vi "setTensao.vi"(6 "delay(ms)":dbl, 7 "Ponto atual":i32, 8 "T.M":dbl caption="Tensão máxima", 9 "P.D.J":dbl, 10 "T.J":dbl caption="Tensão\ndo joelho", 11 "P.A.J":dbl) -> (3 "output voltage":dbl)   [LabVIEW 2012]
uses:
  <instrlib>/Agilent 6XXX Series/Agilent 6XXX Series.lvlib
panel:
  out "error out":errorcluster
  in  "error in (no error)":errorcluster
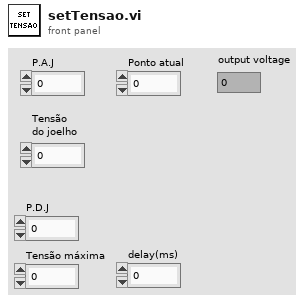
[diagram p1: front panel]
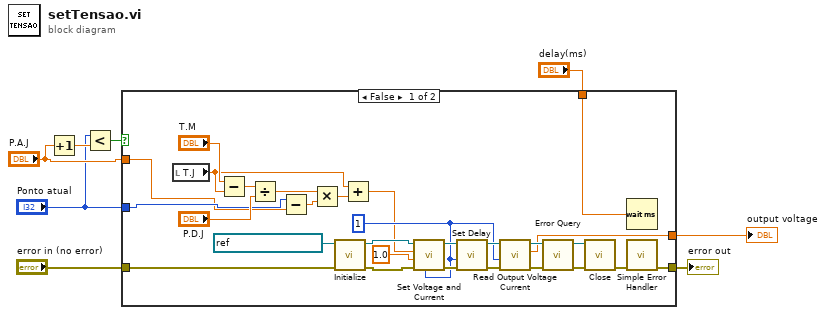
[diagram p0: block diagram]
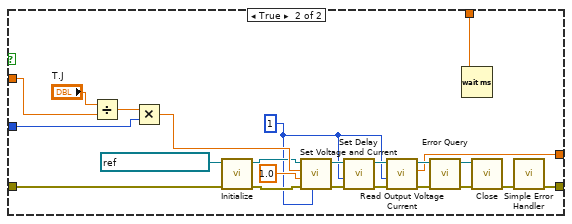
[diagram p2: hidden frame]
diagram:
  n1 = Increment(x="P.A.J") -> (x+1=w7:dbl)
  n2 = Less?(x="Ponto atual", y=w7) -> (x < y?=w8:bool)
  n3 = case shown="False" w8 {
    tunnel: "P.A.J" -> [w14 w59]
    tunnel: "Ponto atual" -> [w15 w58]
    tunnel: [w20 w40] -> w4
    tunnel: [w21 w39] -> w3
    tunnel: "error in (no error)" -> [w22 w38]
    tunnel: "delay(ms)" -> [w19 w37]
    frame False {
      w23 = u8 1 ("channel (1)")
      n4 = local read "T.J"() -> (w10:dbl)
      n5 = Subtract(x="T.M", y=w10) -> (x-y=w17:dbl)
      n6 = Divide(x=w17, y="P.D.J") -> (x/y=w13:dbl)
      n7 = Subtract(x=w15, y=w14) -> (x-y=w12:dbl)
      n8 = Multiply(x=w13, y=w12) -> (x*y=w11:dbl)
      n9 = call <instrlib>:"Initialize.vi"("error in (no error)"=w22, "VISA resource name"=refnum<visa-resource-name> "GPIB0::5::INSTR") -> ("error out"=w28:errorcluster, "VISA resource name out"=w27:refnum<visa-resource-name>)  [unwired: 8 in]
      n10 = Add(x=w10, y=w11) -> (x+y=w9:dbl)
      n11 = call <instrlib>:"Set Voltage and Current.vi"("channel (1)"=w23, "error in (no error)"=w28, "current (0 A)"=1.0, "voltage (0 V)"=w9, "VISA resource name"=w27) -> ("error out"=w31:errorcluster, "VISA resource name out"=w32:refnum<visa-resource-name>)  [unwired: 5 in]
      n12 = call <instrlib>:"Set Delay.vi"("error in (no error)"=w31, "channel (1)"=w23, "VISA resource name"=w32) -> ("error out"=w34:errorcluster, "VISA resource name out"=w33:refnum<visa-resource-name>)  [unwired: 7 in]
      n13 = call <instrlib>:"Read Output Voltage Current.vi"("error in (no error)"=w34, "channel (1)"=w23, "VISA resource name"=w33) -> ("error out"=w29:errorcluster, "output voltage"=w20:dbl, "VISA resource name out"=w30:refnum<visa-resource-name>)  [unwired: 5 in, 1 out]
      n14 = call <instrlib>:"Error Query.vi"("error in (no error)"=w29, "VISA resource name"=w30) -> ("error out"=w25:errorcluster, "VISA resource name out"=w26:refnum<visa-resource-name>)  [unwired: 6 in, 2 out]
      n15 = call <instrlib>:"Close.vi"("error in (no error)"=w25, "VISA resource name"=w26) -> ("error out"=w24:errorcluster)  [unwired: 9 in]
      n16 = Wait (ms)(milliseconds to wait=w19) -> ()  [unwired: 1 out]
      n17 = call <vilib>:"Simple Error Handler.vi"("error in (no error)"=w24) -> ("error out"=w21:errorcluster)  [unwired: 4 in, 4 out]
    }
    frame True {
      w42 = u8 1 ("channel (1)")
      n18 = Divide(x="T.J", y=w59) -> (x/y=w43:dbl)
      n19 = Multiply(x=w43, y=w58) -> (x*y=w53:dbl)
      n20 = call <instrlib>:"Initialize.vi"("error in (no error)"=w38, "VISA resource name"=refnum<visa-resource-name> "GPIB0::5::INSTR") -> ("error out"=w48:errorcluster, "VISA resource name out"=w47:refnum<visa-resource-name>)  [unwired: 8 in]
      n21 = call <instrlib>:"Set Voltage and Current.vi"("channel (1)"=w42, "error in (no error)"=w48, "current (0 A)"=1.0, "voltage (0 V)"=w53, "VISA resource name"=w47) -> ("error out"=w51:errorcluster, "VISA resource name out"=w52:refnum<visa-resource-name>)  [unwired: 5 in]
      n22 = call <instrlib>:"Set Delay.vi"("error in (no error)"=w51, "channel (1)"=w42, "VISA resource name"=w52) -> ("error out"=w55:errorcluster, "VISA resource name out"=w54:refnum<visa-resource-name>)  [unwired: 7 in]
      n23 = call <instrlib>:"Read Output Voltage Current.vi"("error in (no error)"=w55, "channel (1)"=w42, "VISA resource name"=w54) -> ("error out"=w49:errorcluster, "output voltage"=w40:dbl, "VISA resource name out"=w50:refnum<visa-resource-name>)  [unwired: 5 in, 1 out]
      n24 = call <instrlib>:"Error Query.vi"("error in (no error)"=w49, "VISA resource name"=w50) -> ("error out"=w45:errorcluster, "VISA resource name out"=w46:refnum<visa-resource-name>)  [unwired: 6 in, 2 out]
      n25 = Wait (ms)(milliseconds to wait=w37) -> ()  [unwired: 1 out]
      n26 = call <instrlib>:"Close.vi"("error in (no error)"=w45, "VISA resource name"=w46) -> ("error out"=w44:errorcluster)  [unwired: 9 in]
      n27 = call <vilib>:"Simple Error Handler.vi"("error in (no error)"=w44) -> ("error out"=w39:errorcluster)  [unwired: 4 in, 4 out]
    }
  }
  "output voltage" <- w4
  "error out" <- w3
